vi "Configure Trigger Sweep.vi"(8 "error in (no error)":errorcluster, 9 "Trigger Sweep Type (0: Auto)":u16(ring) items=["Auto", "Normal", "Single"], 10 "Trigger Type (0: Edge)":u16(ring) items=["Edge", "Pulse", "Video", "Pattern", "Duration"], 11 "VISA resource name":refnum<visa-resource-name>) -> (0 "error out":errorcluster, 3 "VISA resource name out":refnum<visa-resource-name>)   [LabVIEW 2017, in "RIGOL DS1000 Series.lvlib"]
doc: "Configures trigger sweep type"
uses:
  RIGOL DS1000 Series.lvlib
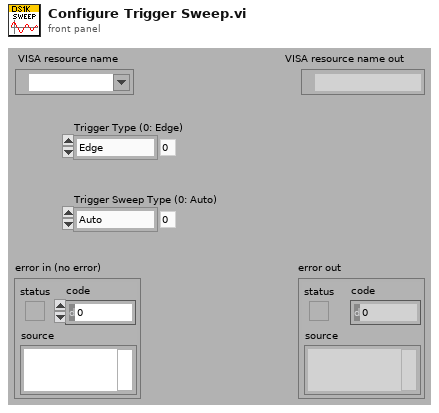
[diagram p1: front panel]
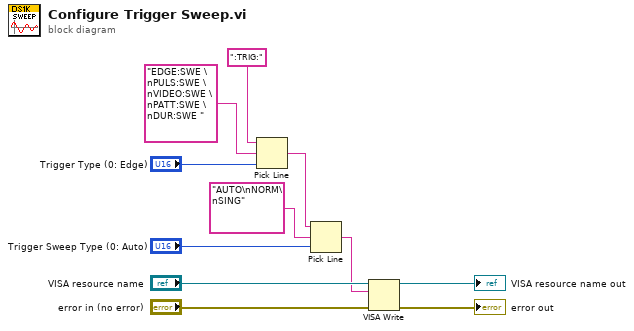
[diagram p0: block diagram]
diagram:
  n1 = Pick Line(string ("")=":TRIG:", multi-line string="EDGE:SWE \nPULS:SWE \nVIDEO:SWE \nPATT:SWE \nDUR:SWE ", line index="Trigger Type (0: Edge)") -> (output string=w6:string)
  n2 = Pick Line(string ("")=w6, multi-line string="AUTO\nNORM\nSING", line index="Trigger Sweep Type (0: Auto)") -> (output string=w3:string)
  n3 = VISA Write(VISA resource name="VISA resource name", write buffer=w3, error in (no error)="error in (no error)") -> (VISA resource name out=→"VISA resource name out":refnum<visa-resource-name>, error out=→"error out":errorcluster)  [unwired: 1 out]
